vi "Display_Console.vi"(8 "error in (no error)":errorcluster) -> (0 "error out":errorcluster)   [LabVIEW 2013]
doc: "This is the display console, It shows the current values of the elevator processes.. [Covers: UI3]"
uses:
  Messaging/Msg_Control.ctl
  Display_Enum.ctl
  Display_Data.ctl
panel:
  out "Emergency":bool
  out "Door Open":bool
  out "Down":bool
  out "Up":bool
  out "Current Floor":u8(knob) scale=1.0..4.0
  out "Timing":dbl
  # "[Covers: UI3C]"
  # "[Covers: UI3A]"
  # "[Covers: UI3D]"
  # "[Covers: UI3B]"
  # "[Covers: UI3E]"
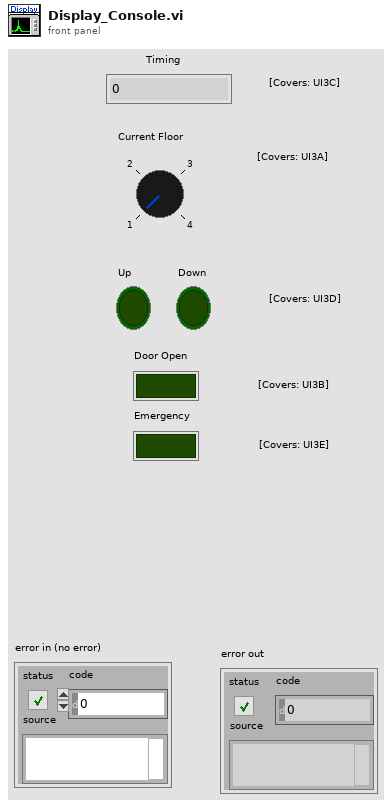
[diagram p1: front panel]
types:
  T1 = typedef "Display_Data.ctl" = cluster{"Timing":dbl, "Current Floor":u8, "Up":bool, "Down":bool, "Door Open":bool, "Emergency":bool}
  T2 = typedef "Display_Enum.ctl" = enum16{"Init", "Update1", "Update2(etc)", "Teminate"}
  T3 = typedef "Msg_Control.ctl" = enum16{"Init_Msg", "Sent_Inits", "Get_Ref", "Close_Ref"}
  T4 = cluster{"queue out":refnum<queue>, "queue out":refnum<queue>, "queue out":refnum<queue>}
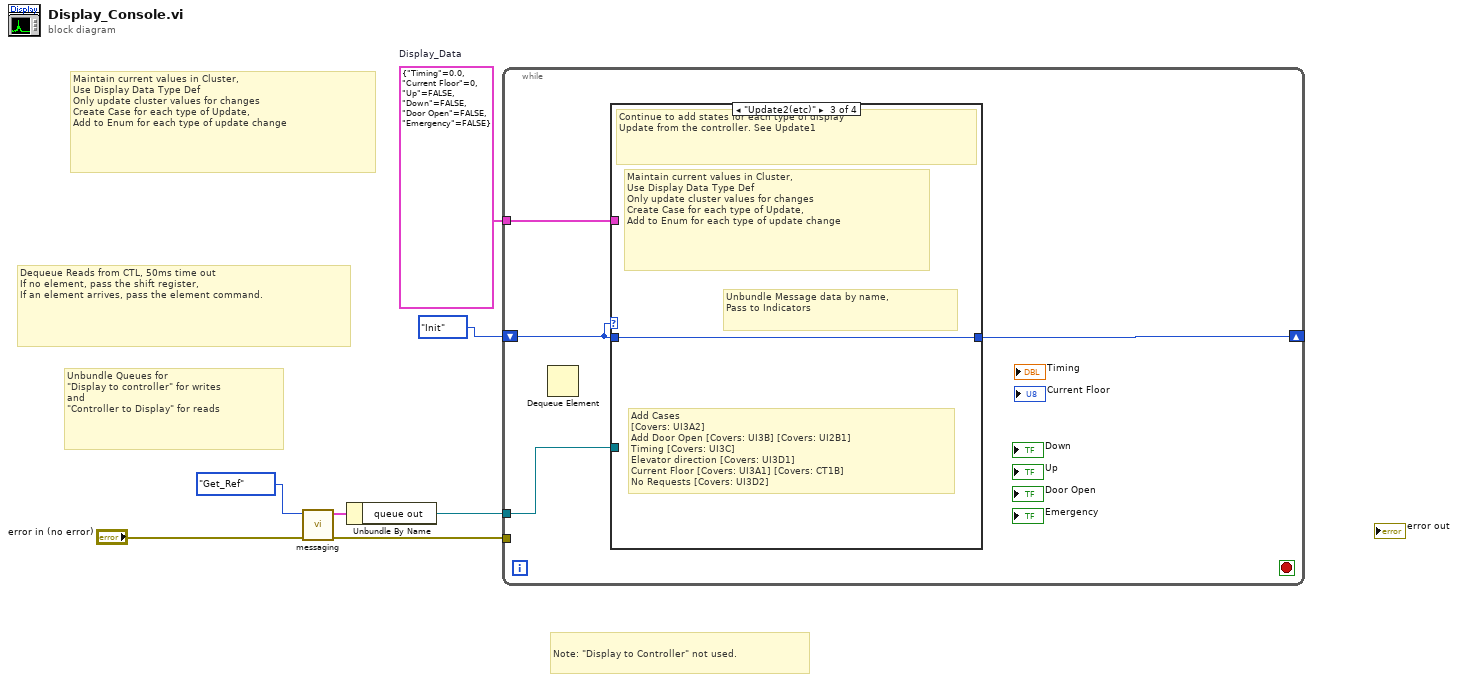
[diagram p0: block diagram]
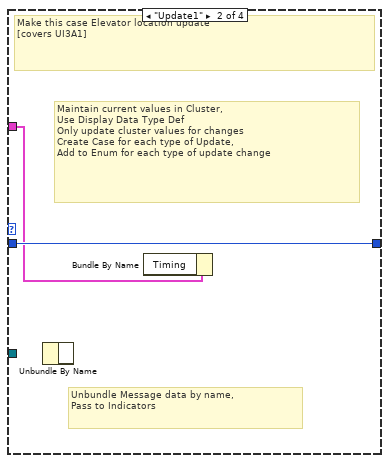
[diagram p3: hidden frame]
diagram:
  w1 = T1 {"Timing"=0.0, "Current Floor"=0, "Up"=FALSE, "Down"=FALSE, "Door Open"=FALSE, "Emergency"=FALSE}  # Display_Data
  # "Maintain current values in Cluster, \nUse Display Data Type Def\nOnly update cluster values for changes\nCreate Case for each type of Update,\nAdd to Enum for each type of update change"
  # "Note: \"Display to Controller\" not used."
  # "Dequeue Reads from CTL, 50ms time out\nIf no element, pass the shift register,\nIf an element arrives, pass the element command."
  # "Unbundle Queues for\n\"Display to controller\" for writes\nand\n\"Controller to Display\" for reads"
  n1 = call "messaging.vi"("error in (no error)"="error in (no error)", "Message_Control"=Msg_Control."Get_Ref") -> ("error out"=w4:errorcluster, "REfs Out"=w6:T4)  [unwired: 8 in]
  n2 = Unbundle By Name(w6) -> ("queue out"=w3:refnum<queue>)
  n3 = while {
    tunnel: w4 -> [_]
    tunnel: w3 -> [w9]
    shift-right: [w10] -> _
    shift-left: Display_Enum."Init" ("Display_Enum") -> [w11]
    tunnel: w1 -> [w8]
    stop <- _ stop-if-true
    n4 = Dequeue Element() -> ()  [unwired: 3 in, 4 out]
    n5 = case shown="\"Update2(etc)\"" w11 {
      tunnel: w11 -> [w12 w14 w15 w16]
      tunnel: [w12 w14 w15 w16] -> w10
      tunnel: w9 -> [_ _ _ _]
      tunnel: w8 -> [_ w13 _ _]
      frame "Init", Default {
        # "[Covers: IS2]"
        # "[Covers: IS2]\nTiming 0.0\nCurrent Floor 0 \nDown F\nUP F\nDoor Open F \nEmergency F"
        # "Pass Values to Inidicators"
        # "Do not use queue data, hardcode init here."
        # "1st queue element is Init, from msg handler"
      }
      frame "Update1" {
        # "Maintain current values in Cluster, \nUse Display Data Type Def\nOnly update cluster values for changes\nCreate Case for each type of Update,\nAdd to Enum for each type of update change"
        # "Unbundle Message data by name, \nPass to Indicators"
        # "Make this case Elevator location update \n[covers UI3A1]"
        n6 = Unbundle By Name() -> ()  [unwired: 1 in, 1 out]
        n7 = Bundle By Name(cluster=w13) -> ()  [unwired: 1 in, 1 out]
      }
      frame "Update2(etc)" {
        # "Add Cases\n[Covers: UI3A2]\nAdd Door Open [Covers: UI3B] [Covers: UI2B1]\nTiming [Covers: UI3C]\nElevator direction [Covers: UI3D1]\nCurrent Floor [Covers: UI3A1] [Covers: CT1B]\nNo Requests [Covers: UI3D2]"
        # "Maintain current values in Cluster, \nUse Display Data Type Def\nOnly update cluster values for changes\nCreate Case for each type of Update,\nAdd to Enum for each type of update change"
        # "Unbundle Message data by name, \nPass to Indicators"
        # "Continue to add states for each type of display \nUpdate from the controller. See Update1"
      }
      frame "Teminate" {
        # "Set timing to 0.0 [Covers: TS5]"
        # "End processes, set indicators, send loop"
      }
    }
  }
